vi "LogData_Http.vi"() -> ()   [LabVIEW 2012, in "LotData.lvclass"]
uses:
  LotData.lvclass
  Controls/TestData.ctl
  Controls/Measurement.ctl
panel:
  in  "Data In":T1 {"50mA Data"."Reverse" format="%#_3g"; "50mA Data"."Current,mA" format="%_6g"; "50mA Data"."Knee Current" format="%#_3g"; "50mA Data"."WL" format="%_6g"; "50mA Data"."Voltage" format="%_6g"; "50mA Data"."Power" format="%_5g"; "20mA Data"."Reverse" format="%#_3g"; "20mA Data"."Current,mA" format="%_6g"; "20mA Data"."Knee Current" format="%#_3g"; "20mA Data"."WL" format="%_6g"; "20mA Data"."Voltage" format="%_6g"; "20mA Data"."Power" format="%_5g"}
  out "Error":bool
  out "LogData_50":string
  in  "50mA Spectra":cluster{"Wavelength":dbl[], "EL Spectrum":dbl[]}
  in  "20mA Spectra":cluster{"Wavelength":dbl[], "EL Spectrum":dbl[]}
  out "LogData":string
  out "LotData out":refnum<class "LotData.lvclass">
  in  "LotData in":refnum<class "LotData.lvclass">
  out "error out":errorcluster
  in  "error in (no error)":errorcluster
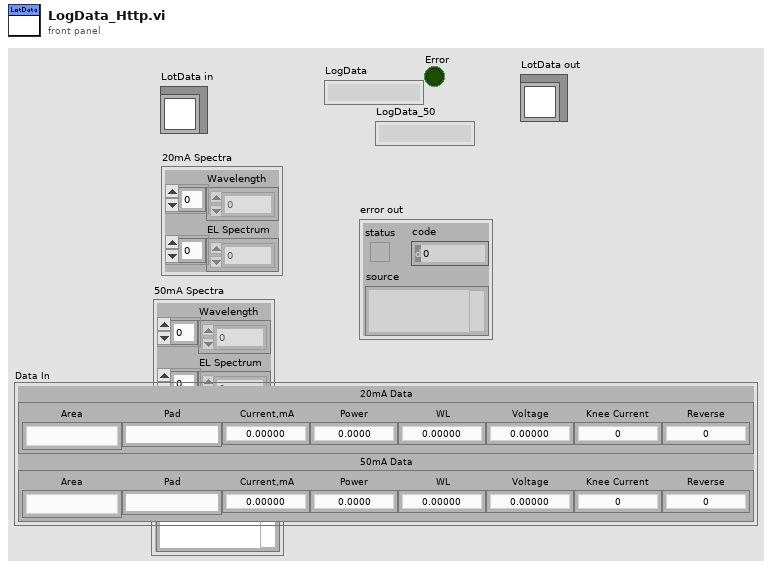
[diagram p1: front panel]
types:
  T1 = typedef "TestData.ctl" = cluster{"20mA Data":T2, "50mA Data ":T2}
  T2 = typedef "Measurement.ctl" = cluster{"Area":string, "Pad":string, "Current,mA":dbl, "Power":dbl, "WL":dbl, "Voltage":dbl, "Knee Current":dbl, "Reverse":dbl}
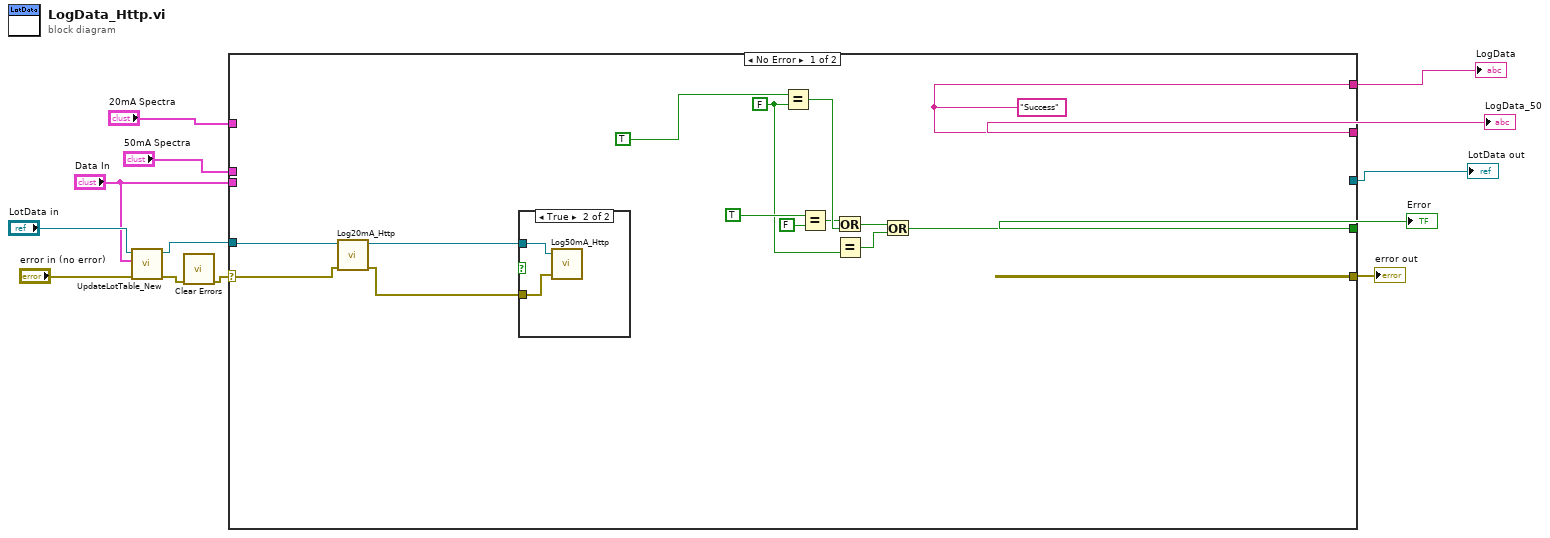
[diagram p0: block diagram]
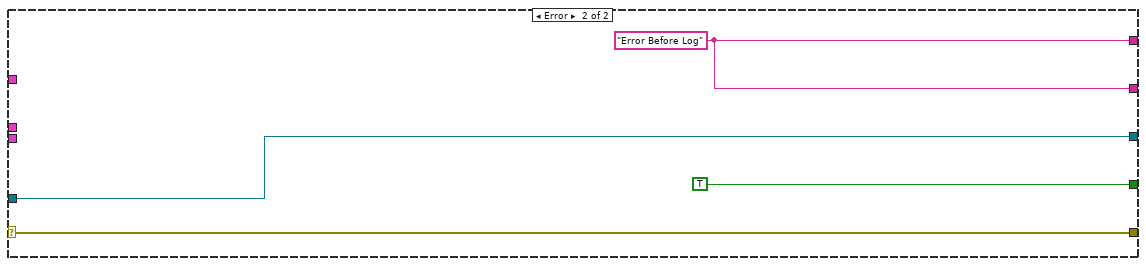
[diagram p3: hidden frame]
diagram:
  n1 = call-dynamic "UpdateLotTable_New.vi"("error in (no error)"="error in (no error)", "input cluster"="Data In", "LotData in"="LotData in") -> ("error out"=w4:errorcluster, "LotData out"=w2:refnum<class "LotData.lvclass">)  [unwired: 7 in]
  n2 = call <vilib>:"Clear Errors.vi"("error in (no error)"=w4) -> ("error out"=w3:errorcluster)  [unwired: 6 in]
  n3 = case shown="No Error" w3 {
    selector: w3 -> [w16 w33]
    tunnel: [_ w33] -> w13
    tunnel: [_ w32] -> w12
    tunnel: w2 -> [w17 w32]
    tunnel: [w22 w31] -> w11
    tunnel: "50mA Spectra" -> [_ _]
    tunnel: "20mA Spectra" -> [_ _]
    tunnel: "Data In" -> [_ _]
    tunnel: [w22 w31] -> w8
    tunnel: [w18 TRUE] -> w7
    frame No Error {
      w22 = "Success" ("LogData")
      w21 = FALSE ("y")
      n4 = call-dynamic "Log20mA_Http.vi"("error in (no error)"=w16, "LotData in"=w17) -> ("error out"=w14:errorcluster, "LotData out"=w15:refnum<class "LotData.lvclass">)  [unwired: 8 in]
      n5 = case shown="True" {
        selector: _ -> [_ _]
        tunnel: w15 -> [_ w29]
        tunnel: w14 -> [_ w28]
        frame False {
        }
        frame True {
          n6 = call "Log50mA_Http.vi"("error in (no error)"=w28, "LotData in"=w29) -> ()  [unwired: 1 in, 3 out]
        }
      }
      n7 = Equal?(x=TRUE, y=w21) -> (x = y?=w24:bool)
      n8 = Equal?(x=TRUE, y=FALSE) -> (x = y?=w23:bool)
      n9 = Or(x=w23, y=w24) -> (x .or. y?=w20:bool)
      n10 = Equal?(y=w21) -> (x = y?=w19:bool)  [unwired: 1 in]
      n11 = Or(x=w20, y=w19) -> (x .or. y?=w18:bool)
    }
    frame Error {
      w31 = "Error Before Log" ("LogData")
    }
  }
  "error out" <- w13
  "LotData out" <- w12
  "LogData" <- w11
  "LogData_50" <- w8
  "Error" <- w7
